vi "digital write.vi"() -> ()   [LabVIEW 2013]
uses:
  <vilib>/LabVIEW Interface for Arduino/Type Defs/Board Type.ctl
  <vilib>/LabVIEW Interface for Arduino/Type Defs/Connection Type.ctl
  <vilib>/LabVIEW Interface for Arduino/Type Defs/Pin Mode.ctl
  <vilib>/LabVIEW Interface for Arduino/LabVIEW Interface for Arduino.lvlib
panel:
  in  "Boolean":bool
  in  "Digital I/O Pin":u8
  in  "stop":bool
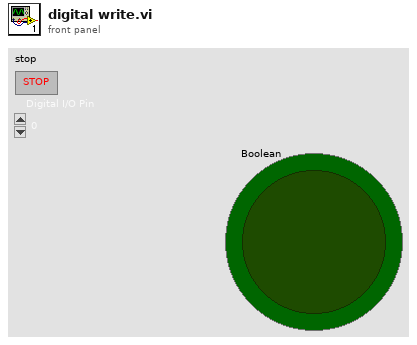
[diagram p1: front panel]
types:
  T1 = typedef "LabVIEW Interface for Arduino.lvlib/Connection Type.ctl" = enum8{"USB / Serial", "XBEE", "BlueSmirf (Bluetooth)"}
  T2 = typedef "LabVIEW Interface for Arduino.lvlib/Board Type.ctl" = enum16{"Uno", "Dimuelanove w/Atmega 328", "Mega 2560"}
  T3 = typedef "LabVIEW Interface for Arduino.lvlib/Arduino Resource.ctl" = cluster{"VISA resource":refnum<visa-resource-name>, "Board Type":T2, "Connection Type":enum8{"USB / Serial"}, "Bytes Per Packet (15)":u8}
  T4 = typedef "LabVIEW Interface for Arduino.lvlib/Pin Mode.ctl" = enum8{"Input", "Output"}
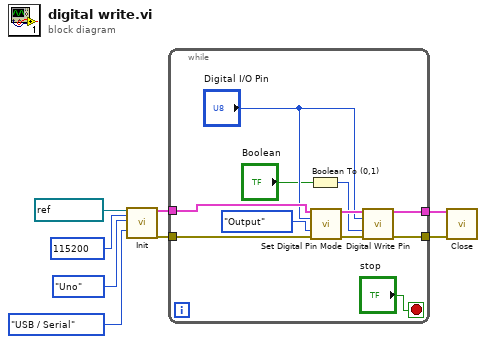
[diagram p0: block diagram]
diagram:
  n1 = call <vilib>:"Init.vi"("VISA resource"=refnum<visa-resource-name> "COM5", "Baud Rate (115200)"=u32 115200, "Board Type (Uno)"=Board_Type."Uno", "Connection Type (USB/Serial)"=Connection_Type."USB / Serial") -> ("Arduino Resource"=w4:T3, "error out"=w2:errorcluster)  [unwired: 14 in]
  n2 = while {
    tunnel: w4 -> [w19]
    tunnel: [w17] -> w3
    tunnel: w2 -> [w16]
    tunnel: [w14] -> w1
    stop <- "stop" stop-if-true
    n3 = Boolean To (0,1)(Boolean="Boolean") -> (0, 1=w9:i16)
    n4 = call <vilib>:"Set Digital Pin Mode.vi"("Arduino Resource"=w19, "Digital I/O Pin"="Digital I/O Pin", "Pin Mode (Input)"=Pin_Mode."Output", "error in"=w16) -> ("Arduino Resource"=w18:T3, "error out"=w15:errorcluster)  [unwired: 10 in]
    n5 = call <vilib>:"Digital Write Pin.vi"("Arduino Resource"=w18, "Digital I/O Pin (0)"="Digital I/O Pin", "Value (0)"=w9, "error in"=w15) -> ("Arduino Resource"=w17:T3, "error out"=w14:errorcluster)  [unwired: 10 in]
  }
  n6 = call <vilib>:"Close.vi"("Arduino Resource"=w3, "error in"=w1) -> ()  [unwired: 13 in, 1 out]
